vi "Query ID.vi"(8 "error in (no error)":errorcluster, 10 "Query String(*IDN?)":string="*IDN?", 11 "DMM in":refnum<class "CS.lvclass">) -> (0 "error out":errorcluster, 2 "ID  string":string, 3 "DMM out":refnum<class "CS.lvclass">)   [LabVIEW 2013, in "CS.lvclass"]
uses:
  Lib.llb/CS.lvclass
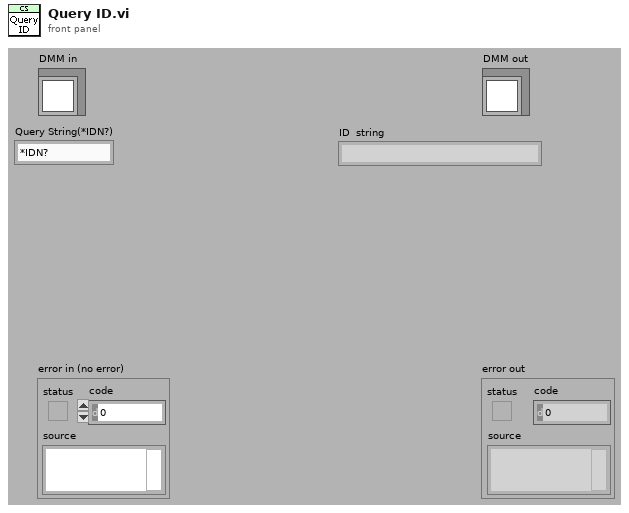
[diagram p1: front panel]
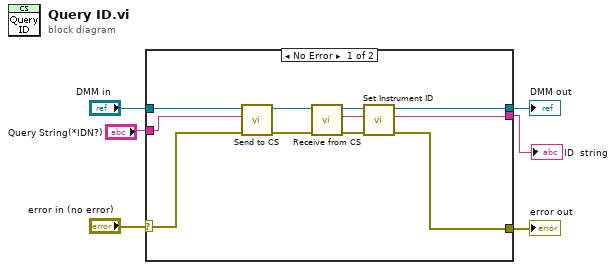
[diagram p0: block diagram]
diagram:
  n1 = case shown="No Error" "error in (no error)" {
    selector: "error in (no error)" -> [w11 w18]
    tunnel: [w15 w18] -> w5
    tunnel: [w16 w17] -> w3
    tunnel: "DMM in" -> [w12 w17]
    tunnel: "Query String(*IDN?)" -> [w8 _]
    tunnel: [w7 _] -> w1
    frame No Error {
      n2 = call-dynamic "Send to CS.vi"("error in (no error)"=w11, "String to write"=w8, "CS in"=w12) -> ("error out"=w13:errorcluster, "CS out"=w14:refnum<class "CS.lvclass">)  [unwired: 7 in]
      n3 = call-dynamic "Receive from CS.vi"("error in (no error)"=w13, "CS in"=w14) -> ("error out"=w9:errorcluster, "Response string"=w7:string, "CS out"=w10:refnum<class "CS.lvclass">)  [unwired: 7 in]
      n4 = call-dynamic "Set Instrument ID.vi"("error in (no error)"=w9, "Instrument ID"=w7, "CS.lvclass in"=w10) -> ("error out"=w15:errorcluster, "CS.lvclass out"=w16:refnum<class "CS.lvclass">)  [unwired: 7 in]
    }
    frame Error {
    }
  }
  "error out" <- w5
  "DMM out" <- w3
  "ID  string" <- w1
